vi "FTW-ActorExtended-LaunchChildActor-Core.vi"(0 "FTW Actor Instance Type":refnum<class "FTW-ActorExtended.lvclass">, 5 "Actor Instance Configuration":string, 11 "error in":errorcluster) -> (4 "FTW Actor Instance":refnum<class "FTW-ActorExtended.lvclass">, 6 "Initialized Response":string, 8 "Instance Inbox Address":string, 10 "Identity":string, 15 "error out":errorcluster)   [LabVIEW 2015, in "FTW-ActorExtended.lvclass"]
uses:
  FTW-ActorExtended.lvclass
  Connector/FTW-ActorConnector.lvclass
  JSON/core/FTW-JSON-Core-EncodingFlags.vi
  JSON/FTW-JSON-Parse.vi
  Reflection/FTW-Reflection-Type.vi
  CodeGen/JSON Deserialize/FTW-JSON-Core-GetFlattenedValue.vi
  CodeGen/JSON Deserialize/FTW-JSON-Deserialize.xnode
panel:
  # "Inputs"
  # "Outputs"
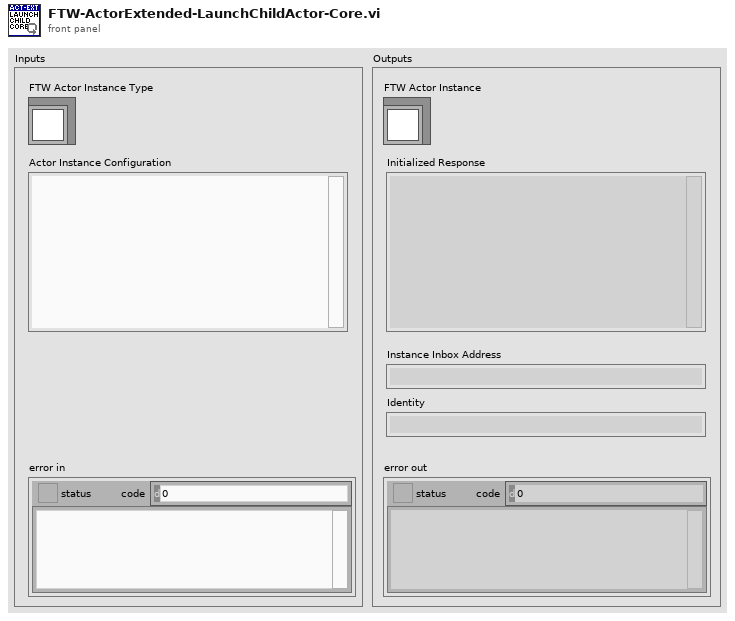
[diagram p1: front panel]
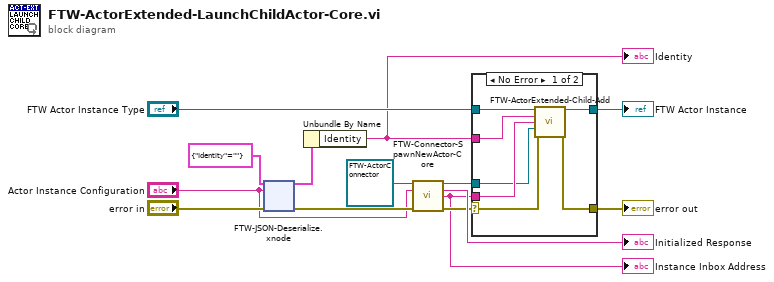
[diagram p0: block diagram]
diagram:
  n1 = xnode "FTW-JSON-Deserialize.xnode"("Type and Defaults"=cluster{"Identity":string} {"Identity"=""}, "JSON String"="Actor Instance Configuration", "error in"="error in") -> ("Values"=w10:cluster{"Identity":string}, "error out"=w6:errorcluster)
  n2 = Unbundle By Name(w10) -> ("Identity"=w1:string)
  "Identity" <- w1
  n3 = call "FTW-Connector-SpawnNewActor-Core.vi"("FTW Actor Connector Type"=refnum<class "FTW-ActorConnector.lvclass"> refnum, "Configuration"="Actor Instance Configuration", "error in"=w6) -> ("FTW Actor Connector"=w2:refnum<class "FTW-ActorConnector.lvclass">, "Initialized Response"=→"Initialized Response":string, "Instance Inbox Address"=w3:string, "error out"=w5:errorcluster)  [unwired: 9 in]
  "Instance Inbox Address" <- w3
  n4 = case shown="No Error" w5 {
    selector: w5 -> [w21 w22]
    tunnel: "FTW Actor Instance Type" -> [w19 w23]
    tunnel: [w18 w23] -> w12
    tunnel: [w20 w22] -> w7
    tunnel: w1 -> [w17 _]
    tunnel: w3 -> [w16 _]
    tunnel: w2 -> [w15 _]
    frame No Error {
      n5 = call "FTW-ActorExtended-Child-Add.vi"("FTW-ActorExtended In"=w19, "Identity"=w17, "Inbox Address"=w16, "Connection"=w15, "error in"=w21) -> ("FTW-ActorExtended Out"=w18:refnum<class "FTW-ActorExtended.lvclass">, "error out"=w20:errorcluster)  [unwired: 9 in]
    }
    frame Error {
    }
  }
  "FTW Actor Instance" <- w12
  "error out" <- w7
